vi "Connect Client.vi"(8 "error in (no error)":errorcluster, 9 "IP Address":string, 10 "Remote Port":u16=1883, 11 "Module ID":i32=-1) -> (0 "error out":errorcluster)   [LabVIEW 2020, in "MQTT_Client.lvlib"]
doc: "Reques to connect the MQTT Client with the given config\n_____\nCreated using Delacor QMH Event Scripter 5.0.0.112."
uses:
  MQTT_Client.lvlib
  Connect Client Argument--cluster.ctl
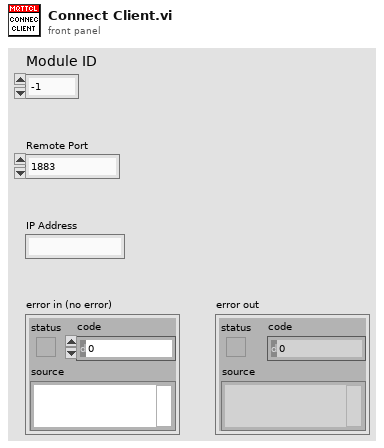
[diagram p1: front panel]
types:
  T1 = typedef "MQTT_Client.lvlib/Connect Client Argument--cluster.ctl" = cluster{"Module ID":i32, "IP Address":string, "Remote Port":u16}
  T2 = typedef "MQTT_Client.lvlib/Request Events--cluster.ctl" = cluster{"Stop Module":refnum<user-event>, "Show Panel":refnum<user-event>, "Hide Panel":refnum<user-event>, "Show Diagram":refnum<user-event>, "Get Module Execution Status":refnum<user-event>, "Connect Client":refnum<user-event>, "Stop Client":refnum<user-event>, "Disconnect":refnum<user-event>, "Subscribe to topic":refnum<user-event>}
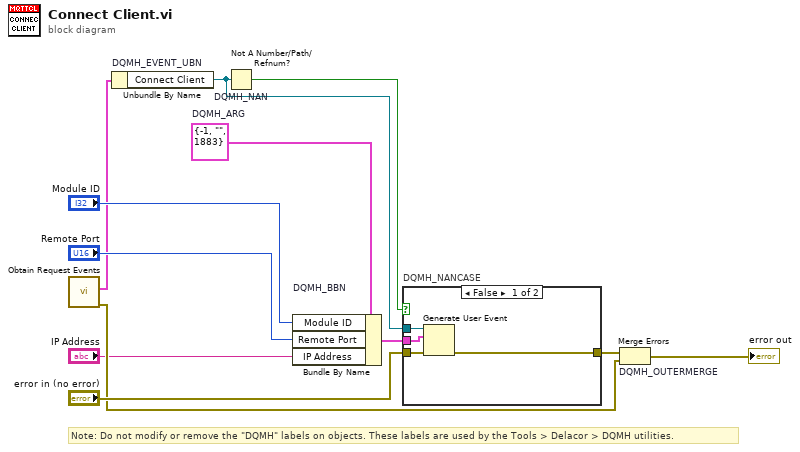
[diagram p0: block diagram]
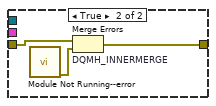
[diagram p2: hidden frame]
diagram:
  w6 = T1 {"Module ID"=-1, "IP Address"="", "Remote Port"=1883}  # DQMH_ARG
  # "Note: Do not modify or remove the \"DQMH\" labels on objects. These labels are used by the Tools > Delacor > DQMH utilities."
  n1 = call "Obtain Request Events.vi"() -> ("error out"=w3:errorcluster, "MQTT_Client Request Events"=w2:T2)  [unwired: 10 in]
  n2 = Unbundle By Name "DQMH_EVENT_UBN"(w2) -> ("Connect Client"=w8:refnum<user-event>)
  n3 = Not A Number/Path/Refnum? "DQMH_NAN"(number/path/refnum=w8) -> (NaN/Path/Refnum?=w9:bool)
  n4 = Bundle By Name "DQMH_BBN"(cluster=w6, "Module ID"="Module ID", "Remote Port"="Remote Port", "IP Address"="IP Address") -> (w10:T1)
  n5 = case "DQMH_NANCASE" shown="False" w9 {
    tunnel: "error in (no error)" -> [w16 w19]
    tunnel: [w15 w18] -> w7
    tunnel: w8 -> [w14 _]
    tunnel: w10 -> [w13 _]
    frame False {
      n6 = Generate User Event(user event=w14, event data cluster=w13, error in=w16) -> (error out=w15:errorcluster)  [unwired: 1 in, 1 out]
    }
    frame True {
      n7 = call "Module Not Running--error.vi"() -> ("error out"=w17:errorcluster)  [unwired: 11 in]
      n8 = Merge Errors "DQMH_INNERMERGE"(w19, w17) -> (w18:errorcluster)
    }
  }
  n9 = Merge Errors "DQMH_OUTERMERGE"(w7, w3) -> (→"error out":errorcluster)
